vi "Transceiver Thread.Set Base Pointer.vi"(8 "error in (no error)":errorcluster, 10 "command parameters":T1, 11 "Transceiver Thread in":refnum<class "Transceiver Thread.lvclass">) -> (0 "error out":errorcluster, 3 "Transceiver Thread out":refnum<class "Transceiver Thread.lvclass">)   [LabVIEW 2017, in "DSF.Engine.lvlib" / "Transceiver Thread.lvclass"]
uses:
  Transceiver Thread.lvclass
  Interface/DSF.Engine.Interface.Transceiver.Command Parameters.ctl
  Interface/DSF.Engine.Interface.Transceiver.Response Data.ctl
  Interface/DSF.Engine.Interface.Transceiver.Response.ctl
  Interface/DSF.Engine.Interface.Transceiver.Response Parameters.ctl
  <vilib>/NI/Memory Manager/Classes/Pointer/Memory.Pointer.lvclass
  <vilib>/NI/Memory Manager/Classes/Pointer/Memory.Pointer.lvclass/Memory.Pointer.ctl
  Transceiver Thread.lvclass/Transceiver Thread.ctl
  <vilib>/NI/Memory Manager/Classes/Pointer/Memory.Pointer.Set Size.vi
  <vilib>/NI/Memory Manager/Classes/Pointer/Memory.Pointer.Set Address.vi
  <vilib>/NI/Memory Manager/Classes/Pointer/Memory.Pointer.Parameter Check.Null Pointer.vi
  <vilib>/NI/Memory Manager/Classes/Pointer/Memory.Pointer.Set Allocated.vi
  <vilib>/NI/Memory Manager/Classes/Pointer/Memory.Pointer.Errors.vi
  <vilib>/NI/Memory Manager/Classes/Pointer/Memory.Pointer.Errors.Null Pointer.vi
  <vilib>/NI/Memory Manager/Classes/Pointer/Memory.Pointer.Get Address.vi
  <vilib>/NI/Memory Manager/Classes/Pointer/Memory.Pointer.Errors.Create Error.vi
  <vilib>/NI/Memory Manager/VIs/New Error Cluster Constant.vi
  <vilib>/NI/Memory Manager/VIs/New Error Cluster Constant (512B).vi
  <vilib>/NI/Memory Manager/VIs/Error Cluster.Set Status.vi
  <vilib>/NI/Memory Manager/VIs/Error Cluster.Set Code.vi
  <vilib>/NI/Memory Manager/VIs/Error Cluster.Set VI Source.vi
  <vilib>/NI/Memory Manager/Constants/Memory.Constants.vi
  <vilib>/NI/Memory Manager/Constants/Memory.Constants.Library Name.vi
  <vilib>/NI/Memory Manager/Classes/Pointer/Memory.Pointer.Errors.Get Info.vi
  <vilib>/NI/Memory Manager/VIs/Source.Write.String.vi
  Interface/DSF.Engine.Interface.Transceiver.lvclass
  Transfer/Transfer Group.lvclass
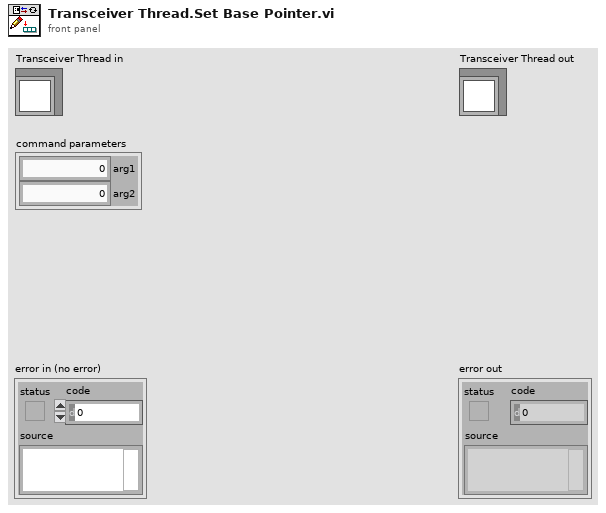
[diagram p1: front panel]
types:
  T1 = typedef "DSF.Engine.lvlib/DSF.Engine.Interface.Transceiver.lvclass/DSF.Engine.Interface.Transceiver.Command Parameters.ctl" = cluster{"arg1":u64, "arg2":u64}
  T2 = typedef "DSF.Engine.lvlib/DSF.Engine.Interface.Transceiver.lvclass/DSF.Engine.Interface.Transceiver.Response Data.ctl" = cluster{"Response":T3, "Response Parameters":T4}
  T3 = typedef "DSF.Engine.lvlib/DSF.Engine.Interface.Transceiver.lvclass/DSF.Engine.Interface.Transceiver.Response.ctl" = enum8{"General Ack", "Shutting Down"}
  T4 = typedef "DSF.Engine.lvlib/DSF.Engine.Interface.Transceiver.lvclass/DSF.Engine.Interface.Transceiver.Response Parameters.ctl" = cluster{"arg1":u64, "arg2":u64}
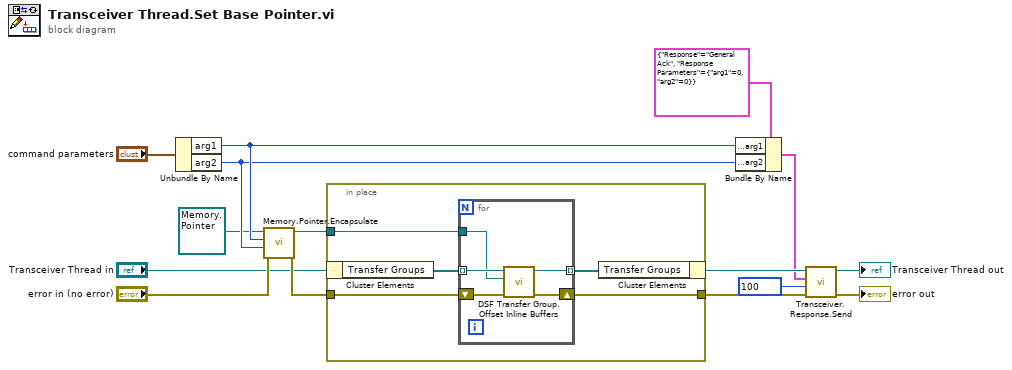
[diagram p0: block diagram]
diagram:
  n1 = Unbundle By Name("command parameters") -> ("arg1"=w5:u64, "arg2"=w4:u64)
  n2 = call <vilib>:"Memory.Pointer.Encapsulate.vi"("error in (no error)"="error in (no error)", "size"=w4, "address"=w5, "Pointer type"=refnum<class "Memory.Pointer.lvclass"> refnum ("Engine Pointer")) -> ("error out"=w6:errorcluster, "Pointer out"=w10:refnum<class "Memory.Pointer.lvclass">)  [unwired: 6 in]
  n3 = in-place {
    in-place-border: w10 -> [w19]
    in-place-border: [w17] -> w9
    in-place-border: w6 -> [w16]
    n4 = in-place-cluster #1("Transceiver Thread in") -> ("Transfer Groups"=w20:refnum<class "Transfer Group.lvclass">[])
    n5 = for {
      tunnel: w20 -> [w25] mode=indexing
      tunnel: w19 -> [w21]
      tunnel: [w24] -> w18 mode=indexing
      shift-right: [w23] -> w17
      shift-left: w16 -> [w22]
      n6 = call "DSF Transfer Group.Offset Inline Buffers.vi"("error in (no error)"=w22, "Engine Pointer"=w21, "Transfer Group in"=w25) -> ("error out"=w23:errorcluster, "Transfer Group out"=w24:refnum<class "Transfer Group.lvclass">)  [unwired: 7 in]
    }
    n7 = in-place-cluster #1("Transfer Groups"=w18) -> (w8:refnum<class "Transceiver Thread.lvclass">)
  }
  n8 = Bundle By Name(cluster=T2 {"Response"=enum."General Ack", "Response Parameters"={"arg1"=0, "arg2"=0}} ("response"), "Response Parameters.arg1"=w5, "Response Parameters.arg2"=w4) -> (w3:T2)
  n9 = call "Transceiver.Response.Send.vi"("error in (no error)"=w9, "timeout in ms (0)"=100, "response"=w3, "Transceiver Thread in"=w8) -> ("error out"=→"error out":errorcluster, "Transceiver Thread out"=→"Transceiver Thread out":refnum<class "Transceiver Thread.lvclass">)  [unwired: 5 in, 1 out]
